vi "Reselect XNET Database Browser.vi"(8 "error in (no error)":errorcluster) -> (0 "error out":errorcluster, 2 "Cancel Out":bool, 3 "XNET Settings":T1={"Database"="", "Cluster"="", "Port"="", "Baud rate [Bd]"=0, "Termination"=0, "CAN I/O Mode"=0, "FD Baud rate [Bd]"=500000, "Priority"=100, "Use Legacy"=FALSE, "FD ISO Mode"=0} {"FD ISO Mode" items=["ISO", "Non ISO", "ISO Legacy"]; "CAN I/O Mode" items=["CAN 2.0", "CAN FD", "CAN FD+BRS"]; "Termination" items=["Off", "On"]})   [LabVIEW 2023, in "Protection and Counter Addon System Explorer.lvlib"]
uses:
  Addon Shared/Types/XNET Settings.ctl
  Protection and Counter Addon System Explorer.lvlib
  <resource>/objmgr/xnet.rc
  Addon Shared/Protection and Counter Addon Shared.lvlib
panel:
  out "CAN I/O Mode":u32(ring) items=["CAN 2.0", "CAN FD", "CAN FD+BRS"]
  in  "Select CAN Cluster":u16(ring) items=["LPA12_C_CANFD_20250319.Cluster"]
  in  "Cancel":bool
  in  "Select":bool
  in  "XNET Database":refnum<k21>
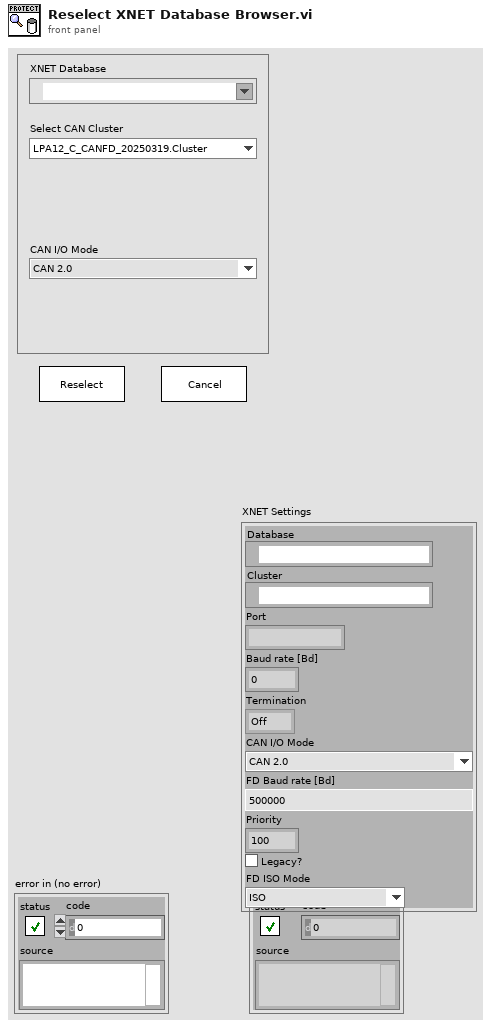
[diagram p1: front panel]
types:
  T1 = typedef "Protection and Counter Addon Shared.lvlib/XNET Settings.ctl" = cluster{"Database":refnum<k21>, "Cluster":refnum<k21>, "Port":string, "Baud rate [Bd]":u64, "Termination":u32, "CAN I/O Mode":u32, "FD Baud rate [Bd]":u64, "Priority":i32, "Use Legacy":bool, "FD ISO Mode":u32}
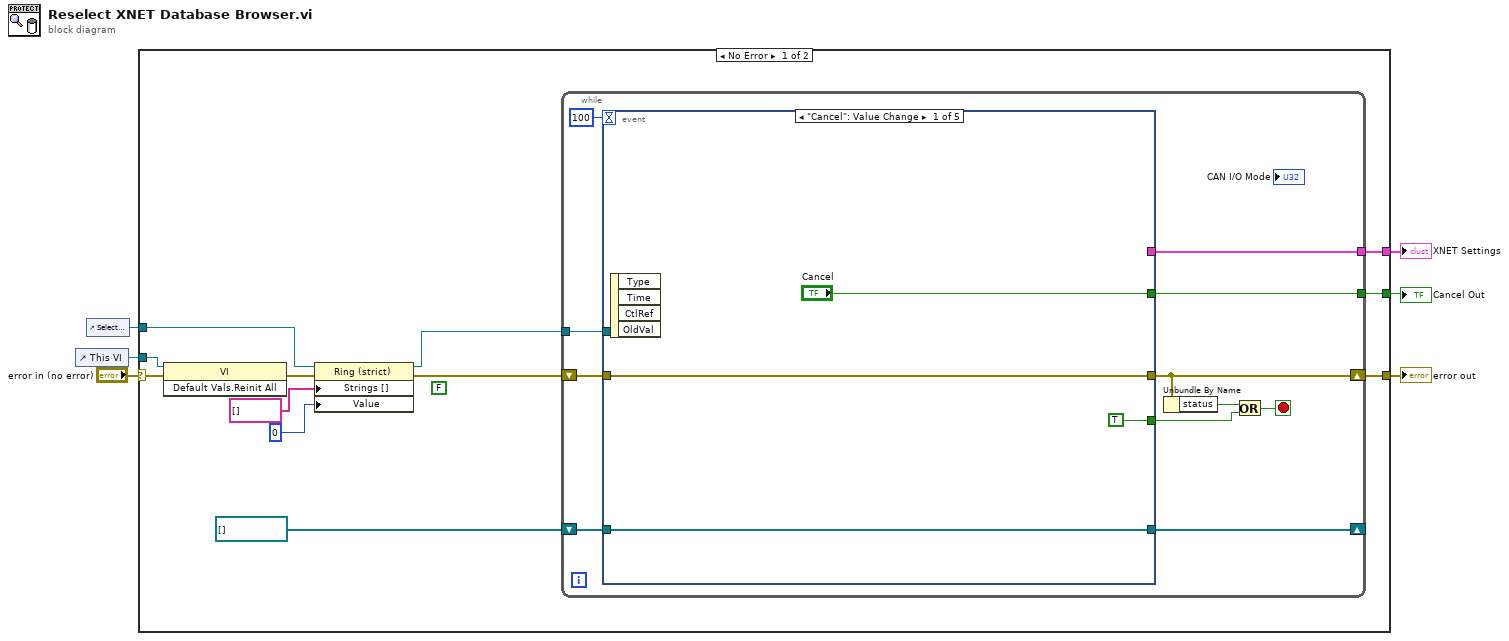
[diagram p0: block diagram]
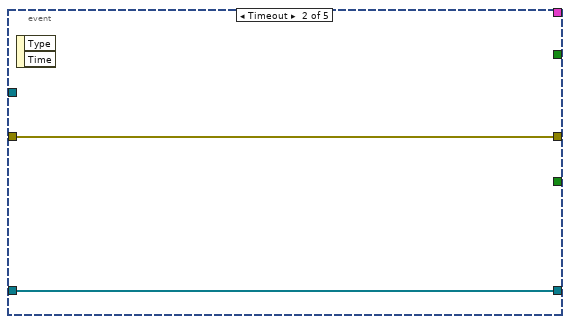
[diagram p2: hidden frame]
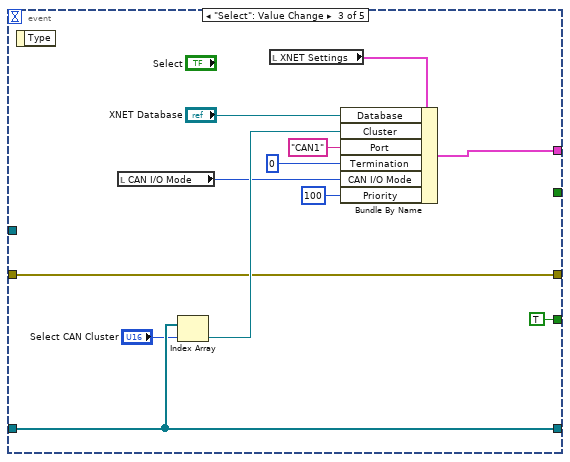
[diagram p3: hidden frame]
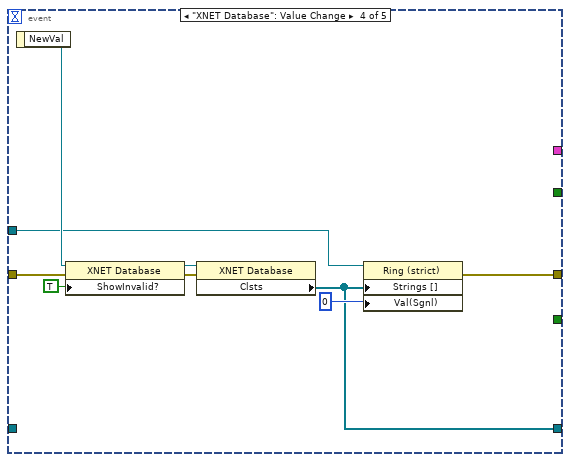
[diagram p4: hidden frame]
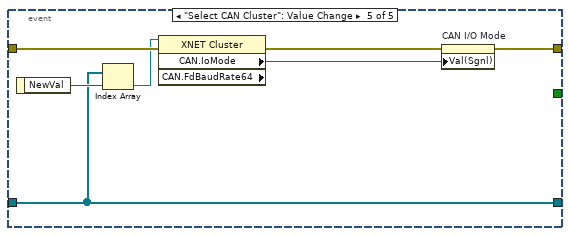
[diagram p5: hidden frame]
diagram:
  n1 = control-ref of="This VI"() -> (w3:refnum<vi>)
  n2 = control-ref of="Select CAN Cluster"() -> (w1:refnum<vi>)
  n3 = case shown="No Error" "error in (no error)" {
    selector: "error in (no error)" -> [w17 w64]
    tunnel: [w15 w64] -> w5
    tunnel: [w18 _] -> w4
    tunnel: w3 -> [w16 _]
    tunnel: [w13 _] -> w2
    tunnel: w1 -> [w12 _]
    frame No Error {
      (unwired) FALSE ("Visible")
      n4 = invoke class="VI" method="Default Vals.Reinit All"(reference=w16, error in=w17) -> (error out=w11:errorcluster)  [unwired: 1 in, 2 out]
      n5 = property on="Property Node" class="Ring (strict)"(reference=w12, error in=w11, "Strings []"=string[] [], "Value"=u16 0) -> (reference out=w10:refnum<vi>, error out=w7:errorcluster)
      n6 = while {
        tunnel: [w29] -> w18
        shift-right: [w27] -> _
        shift-left: refnum<k21>[] [] ("Clsts") -> [w26]
        shift-right: [w23] -> w15
        shift-left: w7 -> [w28]
        tunnel: [w25] -> w13
        tunnel: w10 -> [w19]
        stop <- w20 stop-if-true
        n7 = event shown="[0] \"Cancel\": Value Change" {
          selector: _ -> [_ _ _ _ _]
          dyn-events: _ -> [_ _ _ _ _]
          timeout: 100 -> [_ _ _ _ _]
          tunnel: ["Cancel" _ _ _ _] -> w29
          tunnel: w28 -> [w31 w35 w40 w53 w63]
          tunnel: [w32 w34 w45 w50 w60] -> w27
          tunnel: w26 -> [w32 w34 w45 _ w60]
          tunnel: [w31 w35 w40 w48 w59] -> w23
          tunnel: [_ _ w42 _ _] -> w25
          tunnel: [TRUE _ TRUE _ _] -> w21
          tunnel: w19 -> [_ _ _ w49 _]
          event "Cancel": Value Change {
            n8 = event-data() -> ()  [unwired: 1 in, 4 out]
          }
          event Timeout {
            n9 = event-data() -> ()  [unwired: 1 in, 2 out]
          }
          event "Select": Value Change {
            n10 = event-data() -> ()  [unwired: 1 in, 1 out]
            n11 = local read "CAN I/O Mode"() -> (w36:u32)
            n12 = Index Array(array=w45, index="Select CAN Cluster") -> (element=w43:refnum<k21>)
            n13 = local read "XNET Settings"() -> (w46:T1)
            n14 = Bundle By Name(cluster=w46, "Database"="XNET Database", "Cluster"=w43, "Port"="CAN1", "Termination"=u32 0, "CAN I/O Mode"=w36, "Priority"=100) -> (w42:T1)
          }
          event "XNET Database": Value Change {
            n15 = event-data() -> ("NewVal"=w52:refnum<k21>)  [unwired: 1 in]
            n16 = property class="XNET Database"(reference=w52, error in=w53, "ShowInvalid?"=TRUE ("Show Invalid From Open?")) -> (reference out=w56:refnum<k21>, error out=w55:errorcluster)
            n17 = property class="XNET Database"(reference=w56, error in=w55) -> ("Clsts"=w50:refnum<k21>[])  [unwired: 2 out]
            n18 = property on="Property Node" class="Ring (strict)"(reference=w49, "Strings []"=w50, "Val(Sgnl)"=u16 0 ("Value (Signaling)")) -> (error out=w48:errorcluster)  [unwired: 1 in, 1 out]
          }
          event "Select CAN Cluster": Value Change {
            n19 = event-data() -> ("NewVal"=w62:u16)  [unwired: 1 in]
            n20 = Index Array(array=w60, index=w62) -> (element=w61:refnum<k21>)
            n21 = property class="XNET Cluster" props=["CAN.IoMode", "CAN.FdBaudRate64"](reference=w61, error in=w63) -> (error out=w58:errorcluster, "CAN.IoMode"=w57:u32)  [unwired: 2 out]
            n22 = property on="CAN I/O Mode" class="Ring (strict)"(error in=w58, "Val(Sgnl)"=w57) -> (error out=w59:errorcluster)  [unwired: 1 in, 1 out]
          }
        }
        n23 = Unbundle By Name(w23) -> ("status"=w22:bool)
        n24 = Or(x=w22, y=w21) -> (x .or. y?=w20:bool)
      }
    }
    frame Error {
    }
  }
  "error out" <- w5
  "Cancel Out" <- w4
  "XNET Settings" <- w2
